vi "sub_vi_incertezza_a_b.vi"() -> ()   [LabVIEW 2019]
panel:
  out "Incertezza totale":dbl
  out "Incertezza A":dbl
  out "Incertezza B":dbl
  in  "num misure":dbl
  in  "dev std":dbl
  # "Incertezza A"
  # "Parametri\n\nCella cinese\n0,05 => fs\n\nCella lab\n0,02 => fs\n0,01 => fs\n\nAmplificatore\n0,5 => Avdd / gain\nInput offset drift: 128 => 0.2mV, 64 => 0.4mV\nInput noise: 128 => rate 0 (50nV) e rate Dvdd (90nV)\n\nArduino\nDC: 2 lsb, con freq di clock < 200 kHz.\nEssendo Arduino 1 con freq 16 MHz: clockArduino / prescaler dell'ADC = 125 kHz"
  # "Non linearità\nRipetibilità\nIsteresi"
  # "Incertezza B"
  # "dev std / sqrt(n misurazioni)"
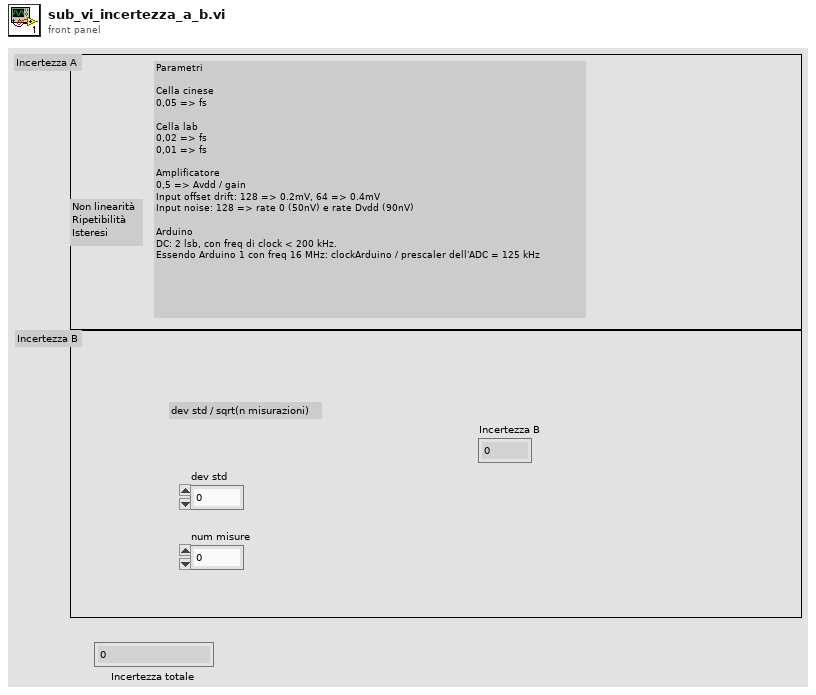
[diagram p1: front panel]
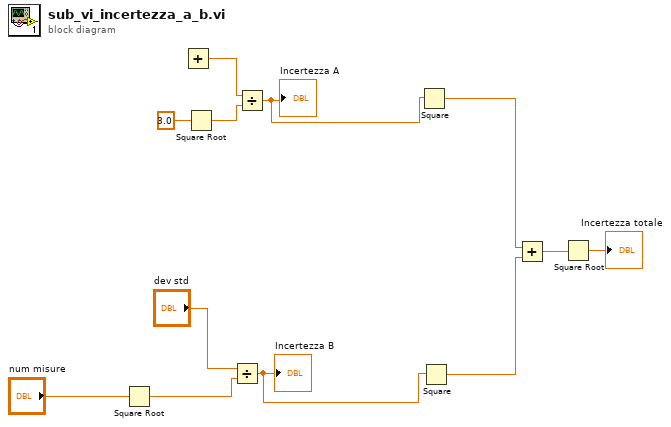
[diagram p0: block diagram]
diagram:
  n1 = Square Root(x="num misure") -> (sqrt(x)=w10:dbl)
  n2 = Add() -> (x+y=w1:dbl)  [unwired: 2 in]
  n3 = Square Root(x=3.0) -> (sqrt(x)=w3:dbl)
  n4 = Divide(x="dev std", y=w10) -> (x/y=w8:dbl)
  "Incertezza B" <- w8
  n5 = Divide(x=w1, y=w3) -> (x/y=w9:dbl)
  "Incertezza A" <- w9
  n6 = Square(x=w9) -> (x^2=w7:dbl)
  n7 = Square(x=w8) -> (x^2=w6:dbl)
  n8 = Add(x=w7, y=w6) -> (x+y=w5:dbl)
  n9 = Square Root(x=w5) -> (sqrt(x)=→"Incertezza totale":dbl)
